vi "RDS Child Subscription.vi"(8 "error in (no error)":errorcluster, 11 "RDS Parent Actor in":refnum<class "RDS Parent Actor.lvclass">) -> (0 "error out":errorcluster, 2 "Subscribed IDs":T1[](array[typedef]), 3 "RDS Parent Actor out":refnum<class "RDS Parent Actor.lvclass">)   [LabVIEW 2015]
uses:
  Libraries/RDS Framework/RDS Message ID.ctl
  Libraries/RDS Framework/RDS Framework.lvlib
  RDS Parent Actor.lvclass
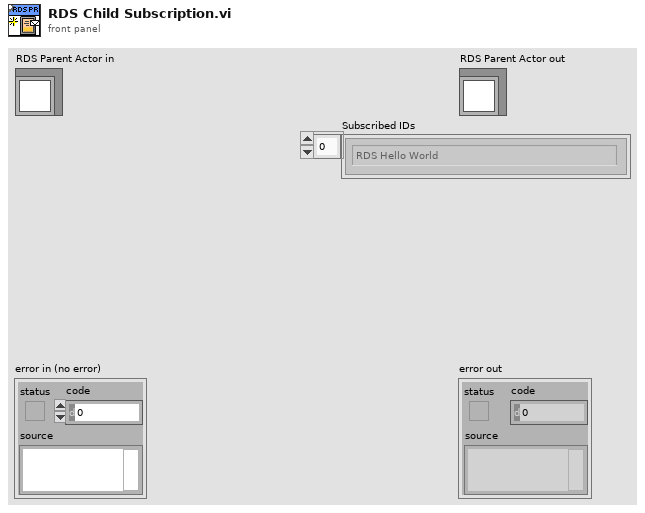
[diagram p1: front panel]
types:
  T1 = typedef "RDS Framework.lvlib/RDS Message ID.ctl" = enum16{"RDS Hello World", "String Message", "AIP_Status", "AIP_Command"}
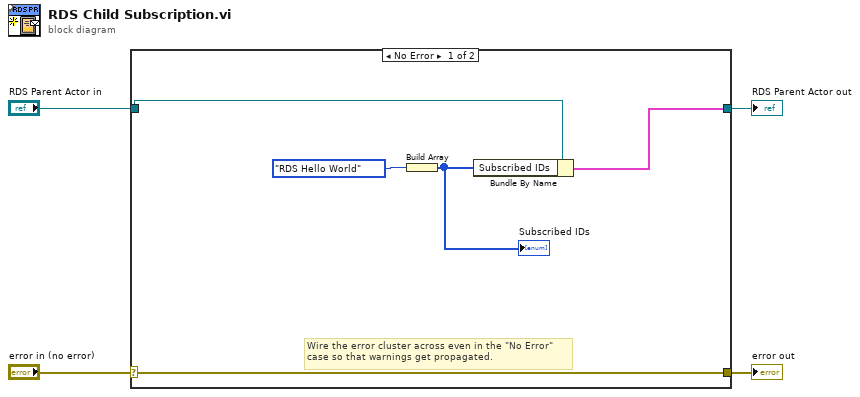
[diagram p0: block diagram]
diagram:
  n1 = case shown="No Error" "error in (no error)" {
    selector: "error in (no error)" -> [w9 w11]
    tunnel: [w9 w11] -> w3
    tunnel: [w5 w10] -> w1
    tunnel: "RDS Parent Actor in" -> [w6 w10]
    frame No Error {
      # "Wire the error cluster across even in the \"No Error\"\ncase so that warnings get propagated."
      n2 = Build Array(RDS_Message_ID."RDS Hello World" ("RDS Message")) -> (w7:T1[])
      "Subscribed IDs" <- w7
      n3 = Bundle By Name(cluster=w6, "Subscribed IDs"=w7) -> (w5:cluster{})
    }
    frame Error {
    }
  }
  "error out" <- w3
  "RDS Parent Actor out" <- w1
